vi "InitialiseClasses.vi"(8 "error in (no error)":errorcluster, 11 "ParseMermaid in":refnum<class "ParseMermaid.lvclass">) -> (0 "error out":errorcluster, 3 "ParseMermaid out":refnum<class "ParseMermaid.lvclass">)   [LabVIEW 2020, in "Mermaid.lvlib" / "ParseMermaid.lvclass"]
uses:
  ParseMermaid.lvclass
  ClassData.ctl
  ClassType.ctl
  Attributes.ctl
  ParseMermaid.lvclass/ParseMermaid.ctl
  <vilib>/regexp/Match Regular Expression.xnode
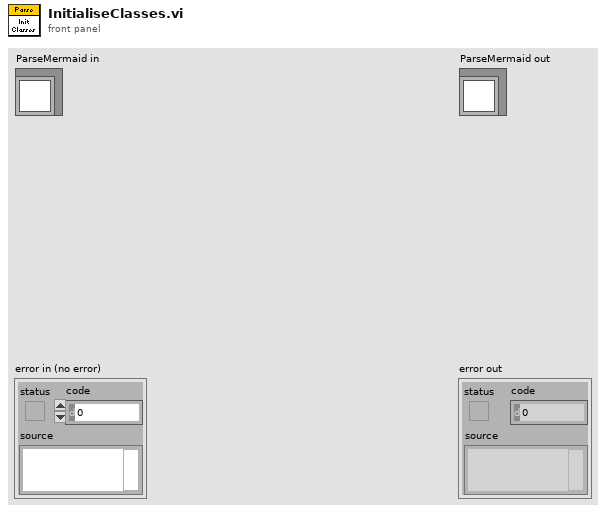
[diagram p1: front panel]
types:
  T1 = typedef "Mermaid.lvlib/ParseMermaid.lvclass/ClassData.ctl" = cluster{"Name":string, "ClassType":T2, "PublicMethods":string[], "PrivateMethods":string[], "FinalPublicAttributes":T3, "FinalPrivateAttributes":T3, "Parent":string}
  T2 = typedef "Mermaid.lvlib/ParseMermaid.lvclass/ClassType.ctl" = enum16{"Interface", "Class"}
  T3 = typedef "Mermaid.lvlib/ParseMermaid.lvclass/Attributes.ctl" = cluster{"Name":string, "Type":i32}[]
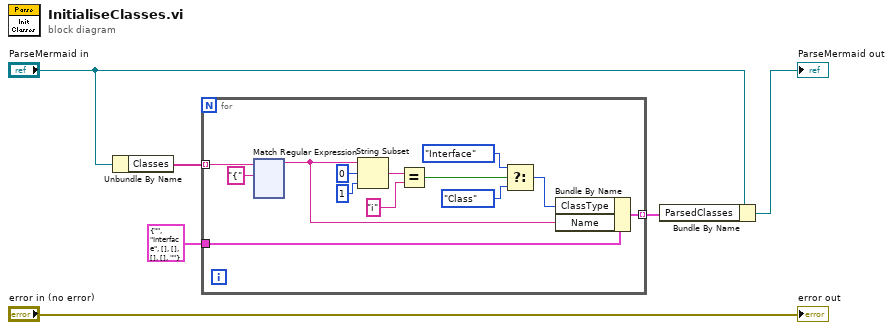
[diagram p0: block diagram]
diagram:
  n1 = Unbundle By Name("ParseMermaid in") -> ("Classes"=w4:string[])
  n2 = for {
    tunnel: w4 -> [w19] mode=indexing
    tunnel: T1 {"Name"="", "ClassType"=enum."Interface", "PublicMethods"=[], "PrivateMethods"=[], "FinalPublicAttributes"=[], "FinalPrivateAttributes"=[], "Parent"=""} ("Class") -> [w7]
    tunnel: [w10] -> w3 mode=indexing
    n3 = xnode "Match Regular Expression"("input string"=w19, "regular expression"="{") -> ("before match"=w11:string)  [unwired: 4 in, 4 out]
    n4 = String Subset(string=w11, offset (0)=0, length (rest)=1 ("length (rest)")) -> (substring=w15:string)
    n5 = Equal?(x=w15, y="i") -> (x = y?=w13:bool)
    n6 = Select(t=ClassType."Interface" ("Enum"), s=w13, f=ClassType."Class" ("Enum")) -> (s? t:f=w12:T2)
    n7 = Bundle By Name(cluster=w7, "ClassType"=w12, "Name"=w11) -> (w10:T1)
  }
  n8 = Bundle By Name(cluster="ParseMermaid in", "ParsedClasses"=w3) -> (→"ParseMermaid out":refnum<class "ParseMermaid.lvclass">)
  "error out" <- "error in (no error)"
